vi "csv_data_upload.vi"(5 "Extra metadata array":T1(array[cluster])=[{"Attribute"="", "Value"="", "Data type"=enum."<null>"}], 6 "Notes":string, 7 "Tags":string, 8 "1D numerical data":dbl[](array[numeric]) format="%0.2f", 9 "2D numerical data":dbl[][](array[numeric]) format="%0.2f", 10 "Name":string, 11 "Parent ID":string="name") -> (0 "error out":errorcluster, 1 "Saved":bool, 2 "body":string, 3 "headers":string)   [LabVIEW 2013]
uses:
  <vilib>/Utility/file.llb/Write To Spreadsheet File (DBL).vi
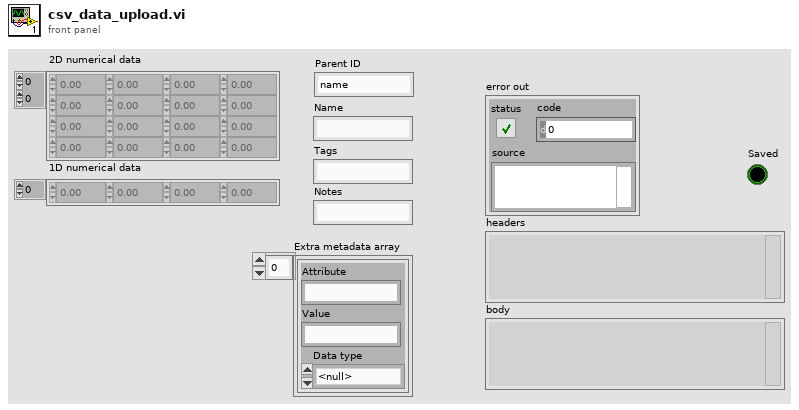
[diagram p1: front panel]
types:
  T1 = cluster{"Attribute":string, "Value":string, "Data type":enum16{"Numeric", "String", "1D array of strings", "1D array of doubles", "Data JSON string", "<null>"}}[]
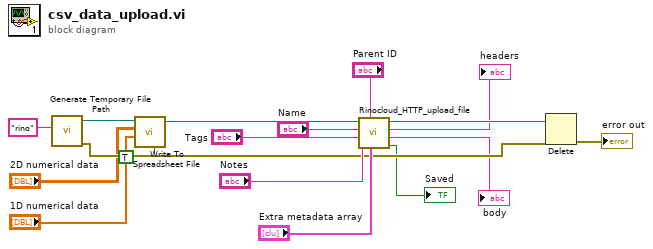
[diagram p0: block diagram]
diagram:
  n1 = call <vilib>:"Generate Temporary File Path.vi"("Temporary File Extension (tmp)"="rino" ("name or relative path")) -> ("error out"=w14:errorcluster, "Unique Temporary File Path"=w11:path)  [unwired: 9 in]
  n2 = call-poly <vilib>:"Write To Spreadsheet File.vi"("transpose? (no:F)"=TRUE, "1D data"="1D numerical data", "2D data"="2D numerical data", "file path (dialog if empty)"=w11) -> ("new file path (Not A Path if cancelled)"=w7:path)  [unwired: 4 in]
  n3 = call "Rinocloud_HTTP_upload_file.vi"("Extra metadata array"="Extra metadata array", "Parent ID"="Parent ID", "Notes"="Notes", "Tags"="Tags", "Name"="Name", "Path"=w7) -> ("Saved"=→"Saved":bool, "body"=→"body":string, "headers"=→"headers":string, "Path out"=w10:path)  [unwired: 1 in, 1 out]
  n4 = Delete(path (use dialog)=w10, error in=w14) -> (error out=→"error out":errorcluster)  [unwired: 3 in, 2 out]
